vi "SetupDMA.vi"(0 "blocks":u32=1, 2 "Drv":u32=1, 3 "pixel":u32=2400, 4 "nos":u32=1) -> (1 "Data Values":u16[][](graph))   [LabVIEW 2015]
uses:
  lv64_eventdriven/board.vis/ESLSCDLL.dll
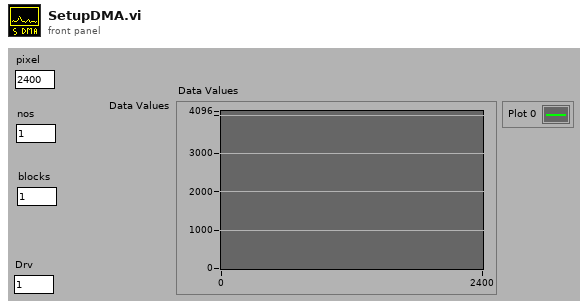
[diagram p1: front panel]
types:
  T1 = enum16{"Init", "Write", "Read array", "Read subarray"}
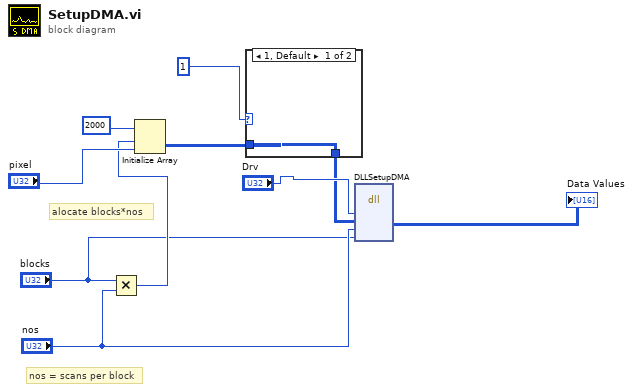
[diagram p0: block diagram]
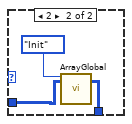
[diagram p2: hidden frame]
diagram:
  # "alocate blocks*nos"
  # "nos = scans per block"
  n1 = Multiply(x="blocks", y="nos") -> (x*y=w6:u32)
  n2 = Initialize Array(u16 2000, w6, "pixel") -> (w3:u16[][])
  n3 = case shown="1, Default" 1 {
    tunnel: w3 -> [w11 w14]
    tunnel: [w11 w13] -> w2
    frame 1, Default {
    }
    frame 2 {
      n4 = call "ArrayGlobal.vi"("Function"=T1."Init", "ArrrayIn"=w14) -> ("ArrayOut"=w13:u16[][])  [unwired: 16 in, 1 out]
    }
  }
  n5 = dll-call lib="C:/ENTW/PCIE/64bit/lv64/lv64_eventdriven/board.vis/ESLSCDLL.dll" fn="DLLSetupDMA" ("lwlscdll.dll:DLLReadFFLoop")("drv"="Drv", "dioden"=w2, "nos"="nos", "blocks"="blocks") -> ("dioden"=→"Data Values":u16[][])  [unwired: 7 in, 2 out]
